vi "Read Dependencies.vi"(8 "error in (no error)":errorcluster, 11 "Transport":refnum<class "Transport.lvclass">) -> (0 "error out":errorcluster, 2 "C.E.":refnum<class "Control Experiment.lvclass">, 3 "Transport":refnum<class "Transport.lvclass">)   [LabVIEW 2019, in "Transport.lvclass"]
uses:
  Transport.lvclass
  Control Experiment/Control Experiment.lvclass
  Transport.lvclass/Transport.ctl
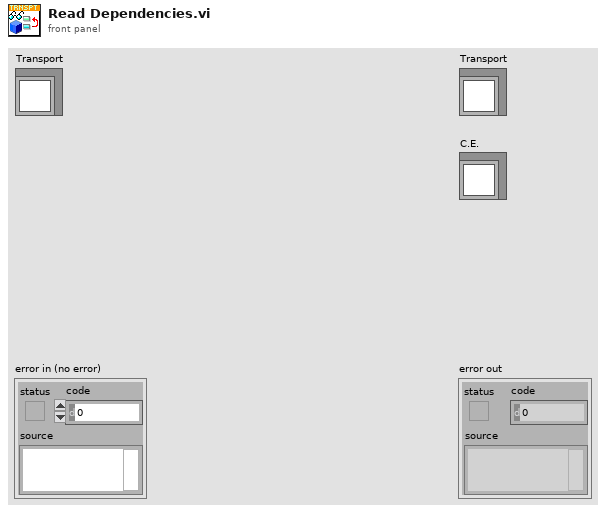
[diagram p1: front panel]
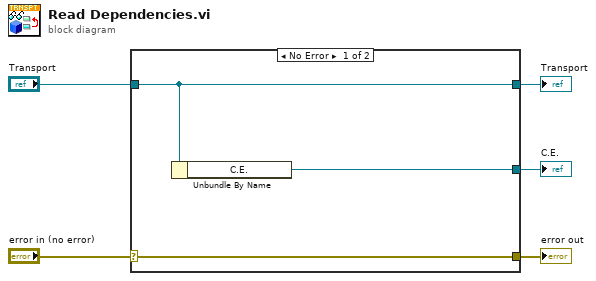
[diagram p0: block diagram]
diagram:
  n1 = case shown="No Error" "error in (no error)" {
    selector: "error in (no error)" -> [w8 w9]
    tunnel: [w8 w9] -> w4
    tunnel: [w7 w10] -> w2
    tunnel: "Transport" -> [w7 w10]
    tunnel: [w6 _] -> w1
    frame No Error {
      n2 = Unbundle By Name(w7) -> ("C.E."=w6:refnum<class "Control Experiment.lvclass">)
    }
    frame Error {
    }
  }
  "error out" <- w4
  "Transport" <- w2
  "C.E." <- w1
